vi "sub_cyclic_prefixer.vi"(8 "FFT size":i32=256, 9 "CP length":i32=64, 11 "time_samples":cdb[](array[numeric])) -> (3 "cp ofdm symbol":cdb[](array[numeric]))   [LabVIEW 2014]
panel:
  out "output size":i32
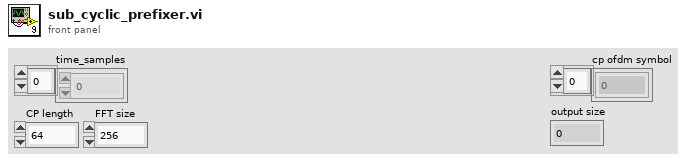
[diagram p1: front panel]
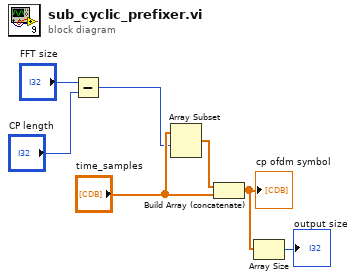
[diagram p0: block diagram]
diagram:
  n1 = Subtract(x="FFT size", y="CP length") -> (x-y=w1:i32)
  n2 = Array Subset(array="time_samples", index=w1) -> (w5:cdb[])  [unwired: 1 in]
  n3 = Build Array (concatenate)(w5, "time_samples") -> (w3:cdb[])
  "cp ofdm symbol" <- w3
  n4 = Array Size(array=w3) -> (size(s)=→"output size":i32)
